vi "2019-05-09_waveform.vi"() -> ()   [LabVIEW 2018]
panel:
  in  "불리언":bool
  out "스윕 차트 3":dbl(graph)
  out "스코프 차트 2":dbl(graph)
  out "스트립 차트":dbl(graph)
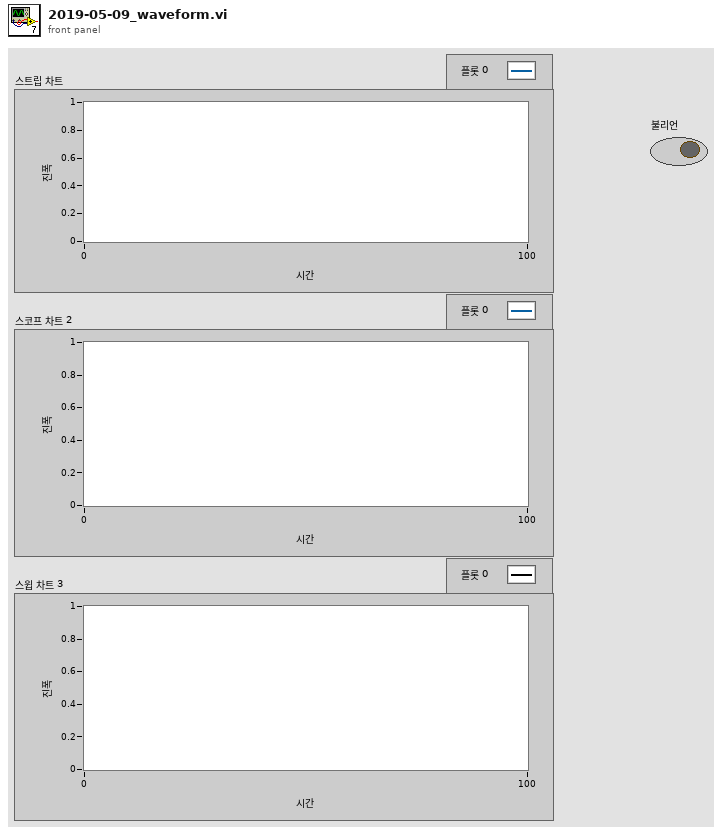
[diagram p1: front panel]
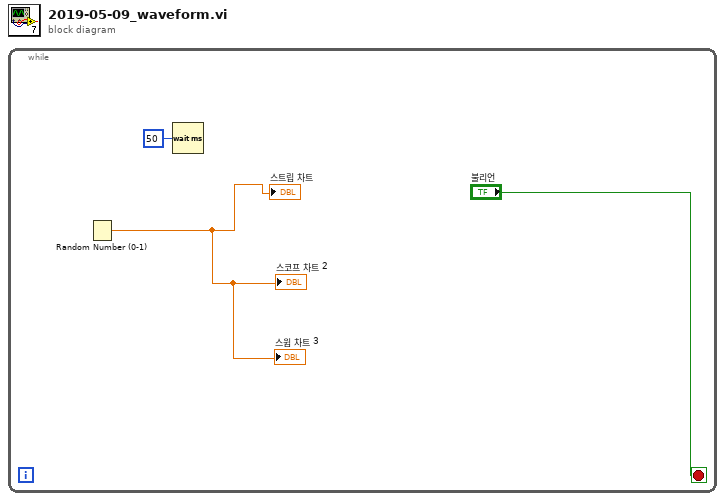
[diagram p0: block diagram]
diagram:
  n1 = while {
    stop <- "불리언" stop-if-true
    n2 = Random Number (0-1)() -> (number: 0 to 1=→"스트립 차트" →"스코프 차트 2" →"스윕 차트 3":dbl)
    n3 = Wait (ms)(milliseconds to wait=u32 50 ("대기 시간 (ms)")) -> ()  [unwired: 1 out]
  }
